vi "GetLogger.vi"(8 "error in (no error)":errorcluster) -> (0 "error out":errorcluster, 3 "Logger":refnum<class "Logger.lvclass">)   [LabVIEW 2014]
uses:
  Logger/Logger.lvclass
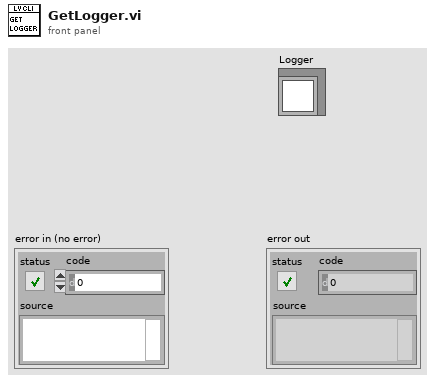
[diagram p1: front panel]
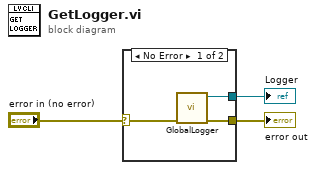
[diagram p0: block diagram]
diagram:
  n1 = case shown="No Error" "error in (no error)" {
    selector: "error in (no error)" -> [w6 w7]
    tunnel: [w5 w7] -> w2
    tunnel: [w4 _] -> w1
    frame No Error {
      n2 = call "GlobalLogger.vi"("error in (no error)"=w6) -> ("error out"=w5:errorcluster, "Logger"=w4:refnum<class "Logger.lvclass">)  [unwired: 9 in]
    }
    frame Error {
    }
  }
  "error out" <- w2
  "Logger" <- w1
